vi "CLD 2  Elapsed Time Express with pause Front Panel.vi"() -> ()   [LabVIEW 2021]
doc: "CLD 2, Challenge Exercise"
panel:
  in  "Reset Button":bool
  out "Elapsed Time (s)":dbl
  out "Time Has Elapsed":bool
  in  "Auto Reset":bool
  in  "Pause Button":bool
  in  "Stop VI":bool
  out "error out":errorcluster
  in  "error in (no error)":errorcluster
  in  "Time Target (s)":dbl=7.0
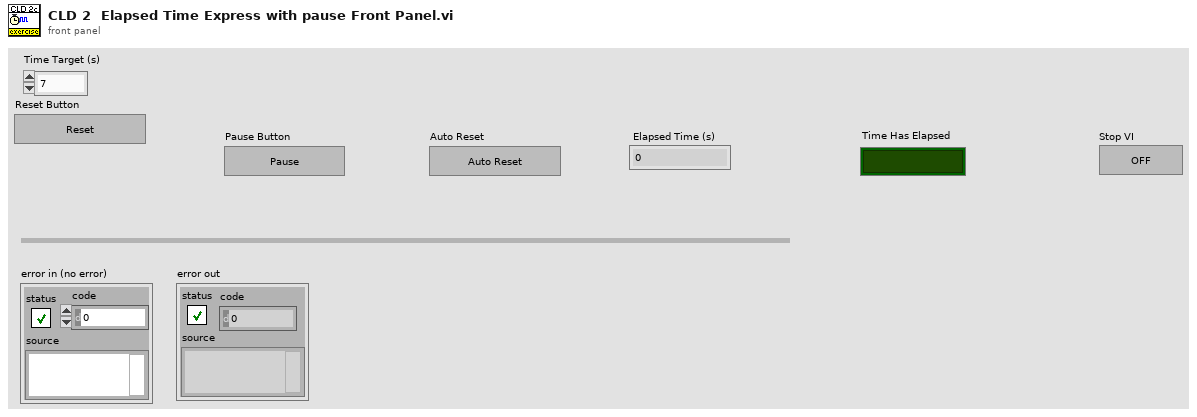
[diagram p1: front panel]
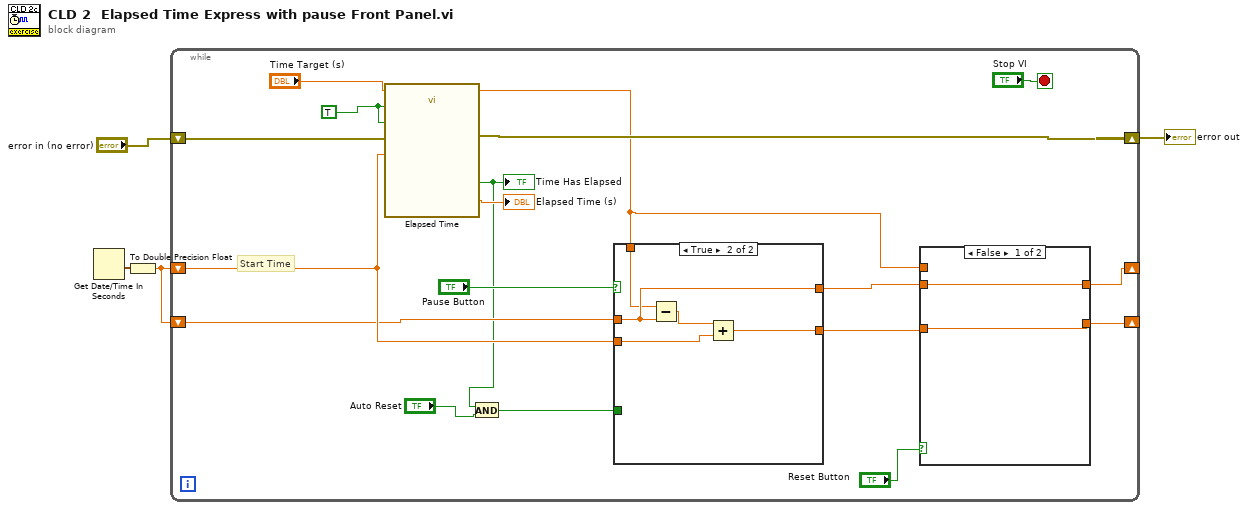
[diagram p0: block diagram]
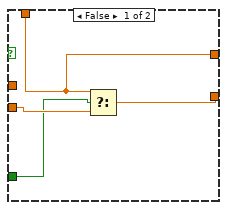
[diagram p3: hidden frame]
diagram:
  n1 = Get Date/Time In Seconds() -> (seconds since 1Jan1904=w2:timestamp)
  n2 = To Double Precision Float(number=w2) -> (double precision float=w1:dbl)
  n3 = while {
    shift-right: [w18] -> w3
    shift-left: "error in (no error)" -> [w19]
    shift-right: [w12] -> _
    shift-left: w1 -> [w16]
    shift-right: [w10] -> _
    shift-left: w1 -> [w15]
    stop <- "Stop VI" stop-if-true
    w5 = TRUE
    # "Start Time"
    n4 = call "Elapsed Time"("Time Target (s)"="Time Target (s)", "Reset"=w5, "Auto Reset"=w5, "error in (no error)"=w19, "Set Start Time (s)"=w16) -> ("Present (s)"=w9:dbl, "Elapsed Time (s)"=→"Elapsed Time (s)":dbl, "Time has Elapsed"=w7:bool, "error out"=w18:errorcluster)  [unwired: 7 in, 4 out]
    "Time Has Elapsed" <- w7
    n5 = And(x=w7, y="Auto Reset") -> (x .and. y?=w6:bool)
    n6 = case shown="True" "Pause Button" {
      tunnel: w9 -> [w27 w30]
      tunnel: w16 -> [w28 w32]
      tunnel: w15 -> [_ w34]
      tunnel: [w27 w34] -> w13
      tunnel: [w29 w31] -> w11
      tunnel: w6 -> [w26 _]
      frame False {
        n7 = Select(t=w27, s=w26, f=w28) -> (s? t:f=w29:dbl)
      }
      frame True {
        n8 = Subtract(x=w30, y=w34) -> (x-y=w33:dbl)
        n9 = Add(x=w33, y=w32) -> (x+y=w31:dbl)
      }
    }
    n10 = case shown="False" "Reset Button" {
      tunnel: [w23 w25] -> w12
      tunnel: w13 -> [w23 _]
      tunnel: [w24 w25] -> w10
      tunnel: w11 -> [w24 _]
      tunnel: w9 -> [_ w25]
      frame False {
      }
      frame True {
      }
    }
  }
  "error out" <- w3
